vi "Functional Imaging-Trial number disabled state.vi"() -> ()   [LabVIEW 2013]
uses:
  Global variables/gl_Functional Imaging-Global variables.vi
panel:
  out "error out":errorcluster
  in  "error in (no error)":errorcluster
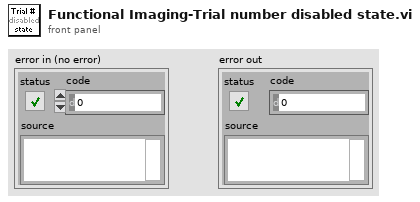
[diagram p1: front panel]
types:
  T1 = enum8{"Enabled", "Disabled", "Disabled and Grayed Out"}
  T2 = typedef "Functional Imging UI Refs.ctl" = cluster{"Menu ref":refnum<k9>, "Image control":refnum<vi>, "VI ref":refnum<vi>, "XGrapher":refnum<vi>, "Smoothing":refnum<vi>, "POI Averaging":refnum<vi>, "Normalize":refnum<vi>, "POI data points in each trial":refnum<vi>, "Channel":refnum<vi>, "Experiment data folder path":refnum<vi>, "[ROI vis]":refnum<vi>, "[Groups] visbl":T3, "Group Name":refnum<vi>, "POI index":refnum<vi>, "Trial No.":refnum<vi>, "Intensity Zoom":refnum<vi>, "Trial Cursor Enabled":refnum<vi>, "Number of Trials (ind 1)":refnum<vi>, "Number of Trials (ind 2)":refnum<vi>, "MiniScans Available":refnum<vi>, "POI Available":refnum<vi>, "Defer graph updates":refnum<vi>, "Waveform selector":refnum<vi>, "#of selected POI":refnum<vi>, "#of selected MiniScans":refnum<vi>, "#of selected groups":refnum<vi>, "Max Z-Projection":refnum<vi>, "Z-Plane Selector":refnum<vi>, "Index of miniscan point to visualise":refnum<vi>, "ROI vis. mode":refnum<vi>, "Total # of points":refnum<vi>, "Index of group clicked on":refnum<vi>, "Pane 1":refnum<vi>, "Pane 2":refnum<vi>, "Pane 3":refnum<vi>, "Pane 4":refnum<vi>, "Pane 5":refnum<vi>, "Pane 6":refnum<vi>, "Deselect all ROI":refnum<vi>, "Deselect all groups":refnum<vi>}
  T3 = typedef "Groups array referecne.ctl" = refnum<vi>
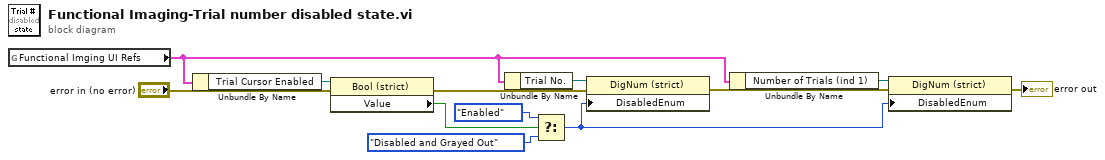
[diagram p0: block diagram]
diagram:
  n1 = global read "gl_Functional Imaging-Global variables.vi" "Functional Imging UI Refs"() -> (w1:T2)
  n2 = Unbundle By Name(w1) -> ("Trial Cursor Enabled"=w8:refnum<vi>)
  n3 = property on="Property Node" class="Bool (strict)"(reference=w8, error in="error in (no error)") -> (error out=w5:errorcluster, "Value"=w7:bool)  [unwired: 1 out]
  n4 = Unbundle By Name(w1) -> ("Trial No."=w9:refnum<vi>)
  n5 = Select(t=T1."Enabled" ("Disabled"), s=w7, f=T1."Disabled and Grayed Out" ("Disabled")) -> (s? t:f=w2:T1)
  n6 = property on="Property Node" class="DigNum (strict)"(reference=w9, error in=w5, "DisabledEnum"=w2) -> (error out=w3:errorcluster)  [unwired: 1 out]
  "error out" <- w3
  n7 = Unbundle By Name(w1) -> ("Number of Trials (ind 1)"=w4:refnum<vi>)
  n8 = property on="Property Node" class="DigNum (strict)"(reference=w4, error in=w3, "DisabledEnum"=w2) -> ()  [unwired: 2 out]
